vi "FINS In-setup.vi"(8 "error i":errorcluster, 10 "msg 3":string, 11 "FINS Header i":T1 {"SNA" max=127 format="%x"; "SA2" max=254 step=1 format="%x"; "SA1" format="%x"; "DA2" max=254 step=1 format="%x"; "DA1" format="%x"; "DNA" max=127 step=1 format="%x"}) -> (0 "error o":errorcluster, 1 "Server Node":u32=10 format="%x", 2 "Client Node":u32=10 format="%x", 3 "FINS Header o":T1 {"SNA" max=127 format="%x"; "SA2" max=254 step=1 format="%x"; "SA1" format="%x"; "DA2" max=254 step=1 format="%x"; "DA1" format="%x"; "DNA" max=127 step=1 format="%x"})   [LabVIEW 2020]
uses:
  FINS/FINS_header.ctl
  FINS/FINS TCP.lvlib
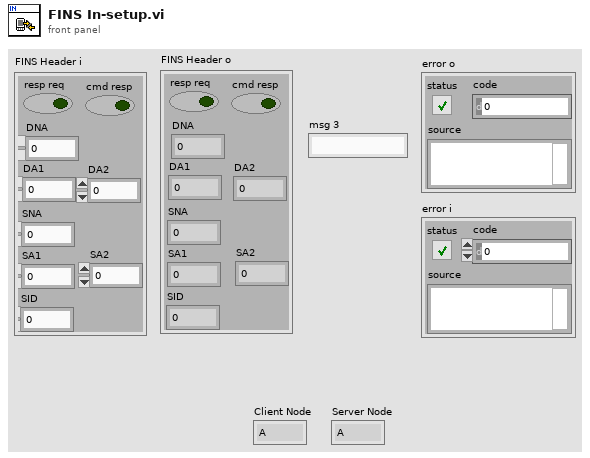
[diagram p1: front panel]
types:
  T1 = typedef "FINS TCP.lvlib/FINS_header.ctl" = cluster{"resp req":bool, "cmd resp":bool, "SID":u8, "DNA":u8, "DA1":u8, "DA2":u8, "SA1":u8, "SA2":u8, "SNA":u8}
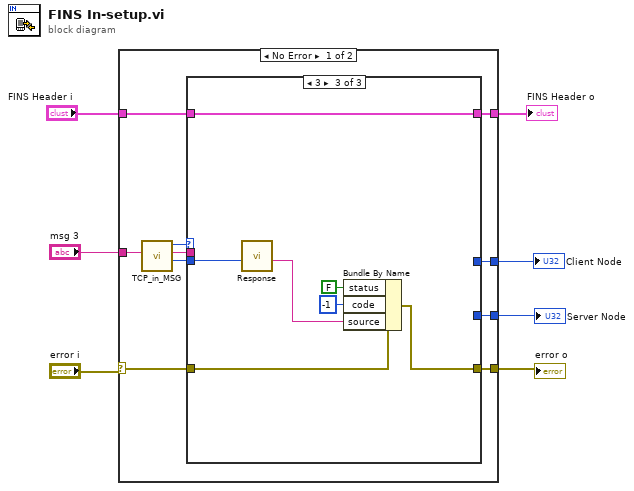
[diagram p0: block diagram]
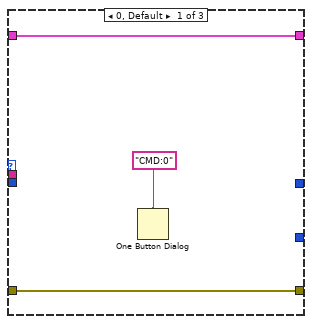
[diagram p2: hidden frame]
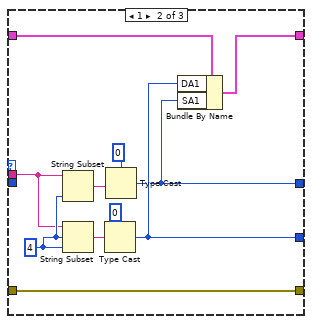
[diagram p3: hidden frame]
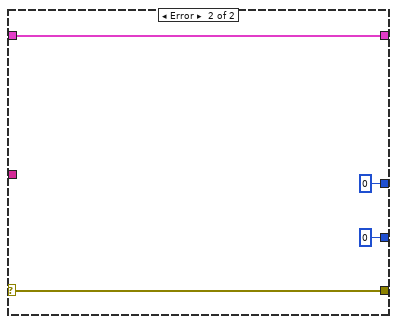
[diagram p4: hidden frame]
diagram:
  n1 = case shown="No Error" "error i" {
    selector: "error i" -> [w12 w42]
    tunnel: "msg 3" -> [w17 _]
    tunnel: [w11 w42] -> w5
    tunnel: "FINS Header i" -> [w15 w41]
    tunnel: [w16 w41] -> w3
    tunnel: [w9 u32 0 ("length")] -> w2
    tunnel: [w8 u32 0 ("length")] -> w1
    frame No Error {
      n2 = call "TCP_in_MSG.vi"("msg i"=w17) -> ("rsp"=w13:u32, "msg o"=w10:string, "cmd"=w14:u32)  [unwired: 8 in]
      n3 = case shown="3" w14 {
        tunnel: [w20 w21 w36] -> w16
        tunnel: w15 -> [w20 w24 w36]
        tunnel: w13 -> [_ _ w38]
        tunnel: w12 -> [w18 w25 w37]
        tunnel: [w18 w25 w35] -> w11
        tunnel: w10 -> [_ w27 _]
        tunnel: [_ w22 _] -> w9
        tunnel: [_ w23 _] -> w8
        frame 0, Default {
          n4 = One Button Dialog(message="CMD:0") -> ()  [unwired: 1 in, 1 out]
        }
        frame 1 {
          w29 = 4 ("length (rest)")
          n5 = String Subset(string=w27, length (rest)=w29) -> (substring=w31:string)  [unwired: 1 in]
          n6 = String Subset(string=w27, offset (0)=w29, length (rest)=w29) -> (substring=w30:string)
          n7 = Type Cast(type=u32 0 ("length"), x=w30) -> (*(type *) &x=w23:u32)
          n8 = Type Cast(type=u32 0 ("length"), x=w31) -> (*(type *) &x=w22:u32)
          n9 = Bundle By Name(cluster=w24, "DA1"=w23, "SA1"=w22) -> (w21:T1)
        }
        frame 3 {
          n10 = call "Response.vi"("rsp"=w38) -> ("error"=w32:string)  [unwired: 10 in]
          n11 = Bundle By Name(cluster=w37, "status"=FALSE, "code"=-1, "source"=w32) -> (w35:errorcluster)
        }
      }
    }
    frame Error {
    }
  }
  "FINS Header o" <- w3
  "error o" <- w5
  "Server Node" <- w1
  "Client Node" <- w2
